vi "Temporised Pop-up Window - Core.vi"(6 "error window":bool, 8 "error constant":errorcluster, 10 "Timeout":dbl, 11 "String":string) -> (0 "error out":errorcluster)   [LabVIEW 2026, in "TALOS.lvlib"]
doc: "Use this VI to create a pop up window that will close if the user press \"OK\" or after the timeout you specify. It is very useful to be sure that an unattended VI will never get blocked because the user is not looking at the screen.\nThe timeout is limited between 1 s and 30 s."
uses:
  TALOS.lvlib
  Global Memory.vi
panel:
  out "self-destroy":u8=5 format="%2.0f"
  in  "Hide errror windows":bool
  out "String out":string
  in  "OK":bool
  # "This message will self-destroy in"
  # "seconds."
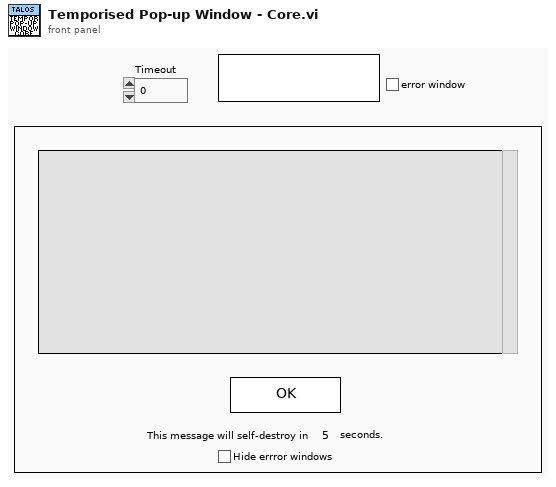
[diagram p1: front panel]
types:
  T1 = enum32{"Invalid", "Standard", "Closed", "Hidden", "Minimized", "Maximized"}
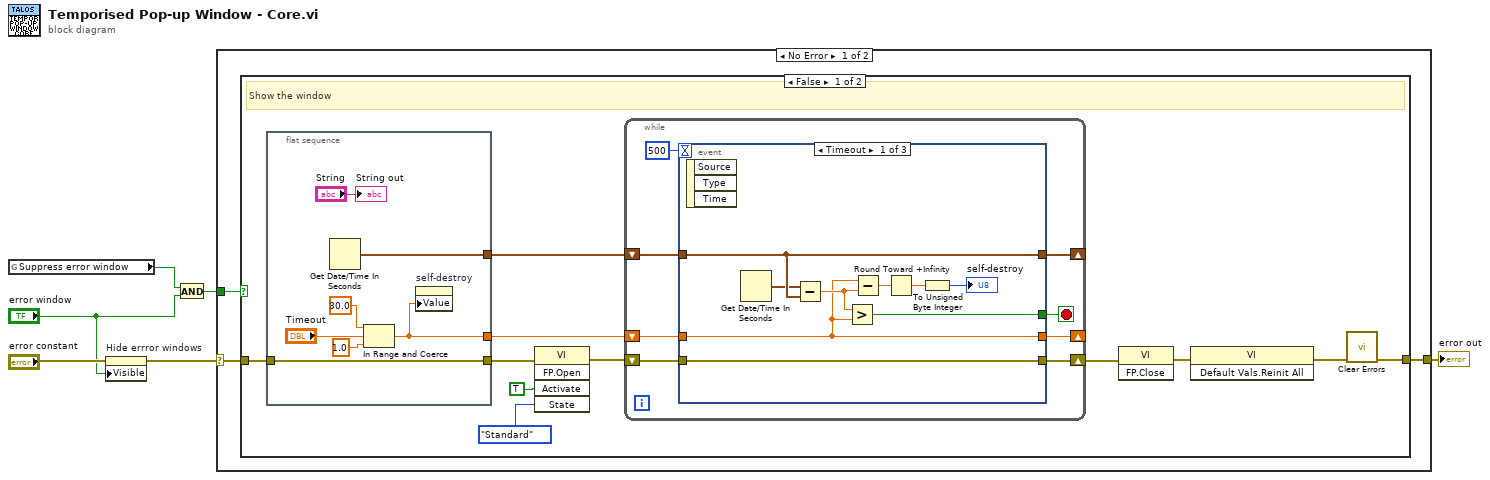
[diagram p0: block diagram]
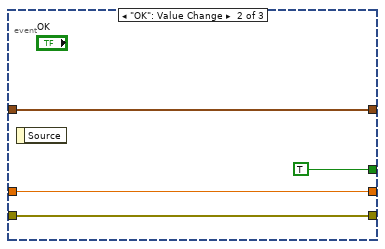
[diagram p2: hidden frame]
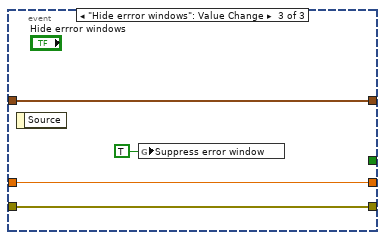
[diagram p3: hidden frame]
diagram:
  n1 = global read "Global Memory.vi" "Suppress error window"() -> (w3:bool)
  n2 = property on="Hide errror windows" class="Bool (strict)"(error in="error constant", "Visible"="error window") -> (error out=w2:errorcluster)  [unwired: 1 in, 1 out]
  n3 = And(x=w3, y="error window") -> (x .and. y?=w1:bool)
  n4 = case shown="No Error" w2 {
    selector: w2 -> [w8 w54]
    tunnel: [w9 w54] -> w6
    tunnel: w1 -> [w7 _]
    frame No Error {
      n5 = case shown="False" w7 {
        tunnel: [w17 w53] -> w9
        tunnel: w8 -> [w14 w53]
        frame False {
          # "Show the window"
          n6 = flat-sequence {
            tunnel: [w27] -> w20
            tunnel: [w25] -> w11
            tunnel: w14 -> [w25]
            tunnel: [w22] -> w18
            frame #0 {
              n7 = Get Date/Time In Seconds() -> (seconds since 1Jan1904=w27:timestamp)
              n8 = In Range and Coerce(upper limit=30.0, x="Timeout", lower limit=1.0) -> (coerced(x)=w22:dbl)  [unwired: 1 out]
              n9 = property on="self-destroy" class="DigNum (strict)"("Value"=w22) -> ()  [unwired: 2 in, 2 out]
              "String out" <- "String"
            }
          }
          n10 = invoke class="VI" method="FP.Open"(error in=w11, "Activate"=TRUE ("Activate?"), "State"=T1."Standard") -> (error out=w10:errorcluster)  [unwired: 2 in, 4 out]
          n11 = while {
            shift-right: [w32] -> _
            shift-left: w20 -> [w33]
            shift-right: [w30] -> w19
            shift-left: w10 -> [w31]
            shift-right: [w28] -> _
            shift-left: w18 -> [w29]
            stop <- w34 stop-if-true
            n12 = event shown="[0] Timeout" {
              selector: _ -> [_ _ _]
              dyn-events: _ -> [_ _ _]
              timeout: 500 -> [_ _ _]
              tunnel: [w42 TRUE _] -> w34
              tunnel: w33 -> [w44 w45 w52]
              tunnel: [w44 w45 w52] -> w32
              tunnel: w31 -> [w41 w47 w50]
              tunnel: [w41 w47 w50] -> w30
              tunnel: w29 -> [w39 w46 w51]
              tunnel: [w39 w46 w51] -> w28
              event Timeout {
                n13 = event-data() -> ()  [unwired: 1 in, 3 out]
                n14 = Get Date/Time In Seconds() -> (seconds since 1Jan1904=w43:timestamp)
                n15 = Subtract(x=w43, y=w44) -> (x-y=w40:dbl)
                n16 = Greater?(x=w40, y=w39) -> (0:w42:bool)
                n17 = Subtract(x=w39, y=w40) -> (x-y=w37:dbl)
                n18 = Round Toward +Infinity(x=w37) -> (ceil(x): smallest int >= x=w36:dbl)
                n19 = To Unsigned Byte Integer(number=w36) -> (unsigned 8bit integer=→"self-destroy":u8)
              }
              event "OK": Value Change {
                n20 = event-data() -> ()  [unwired: 1 in, 1 out]
              }
              event "Hide errror windows": Value Change {
                n21 = event-data() -> ()  [unwired: 1 in, 1 out]
                n22 = global write "Global Memory.vi" "Suppress error window"(TRUE ("Suppress error window")) -> ()
              }
            }
          }
          n23 = invoke class="VI" method="FP.Close"(error in=w19) -> (error out=w16:errorcluster)  [unwired: 2 in, 2 out]
          n24 = invoke class="VI" method="Default Vals.Reinit All"(error in=w16) -> (error out=w15:errorcluster)  [unwired: 2 in, 2 out]
          n25 = call <vilib>:"Clear Errors.vi"("error in (no error)"=w15) -> ("error out"=w17:errorcluster)  [unwired: 5 in, 1 out]
        }
        frame True {
          # "Error window suppressed, do nothing"
        }
      }
    }
    frame Error {
    }
  }
  "error out" <- w6
